vi "buf.vi"() -> ()   [LabVIEW 2012]
panel:
  out "布尔 2":bool
  out "布尔":bool
  in  "停止":bool
  out "波形图表 2":dbl(graph)
  out "波形图表":dbl(graph)
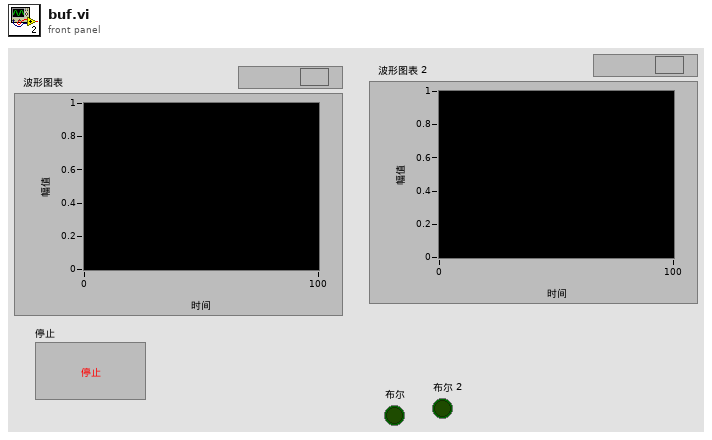
[diagram p1: front panel]
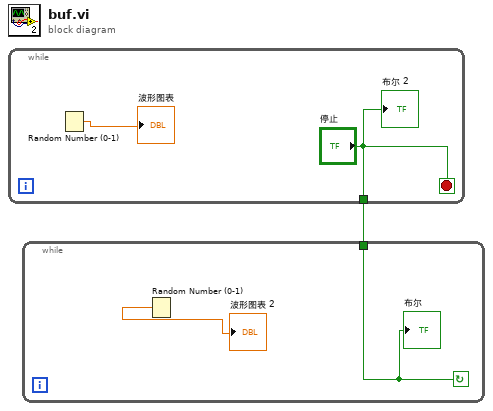
[diagram p0: block diagram]
diagram:
  n1 = while {
    tunnel: ["停止"] -> w1
    stop <- "停止" stop-if-true
    n2 = Random Number (0-1)() -> (number: 0 to 1=→"波形图表":dbl)
    "布尔 2" <- "停止"
  }
  n3 = while {
    tunnel: w1 -> [w4]
    stop <- w4 continue-if-true
    n4 = Random Number (0-1)() -> (number: 0 to 1=→"波形图表 2":dbl)
    "布尔" <- w4
  }
